vi "FGV Laser.vi"(8 "error in (no error)":errorcluster, 10 "FGV Laser Data In":T1 {"Pulse Picker Set" items=["80"=80, "40"=40, "20"=20, "10"=10, "0"=0]}, 11 "Action":T3=enum."Connect") -> (0 "error out":errorcluster, 3 "FGV Laser Data Out":T1 {"Pulse Picker Set" items=["80"=80, "40"=40, "20"=20, "10"=10, "0"=0]})   [LabVIEW 2017]
uses:
  Action Laser.ctl
  FGV Laser Data.ctl
  PulsePickerValues.ctl
  <vilib>/Instr/_visa.llb/VISA Configure Serial Port (Instr).vi
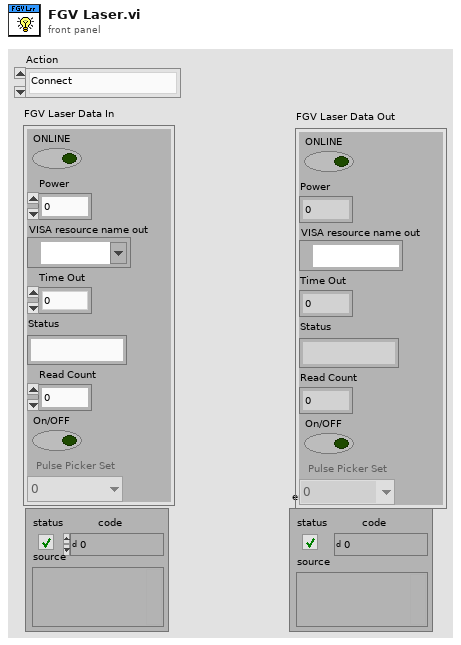
[diagram p1: front panel]
types:
  T1 = typedef "FGV Laser Data.ctl" = cluster{"ONLINE":bool, "Power":dbl, "VISA resource name out":refnum<visa-resource-name>, "Time Out":dbl, "Status":string, "Read Count":u32, "On/OFF":bool, "Pulse Picker Set":T2}
  T2 = typedef "PulsePickerValues.ctl" = u16
  T3 = typedef "Action Laser.ctl" = enum16{"Initialize", "Connect", "Disconnect", "Set Power", "Get Power", "Set Pulse Picker", "Get Pulse Picker", "Laser ON", "Laser OFF", "Read Visa"}
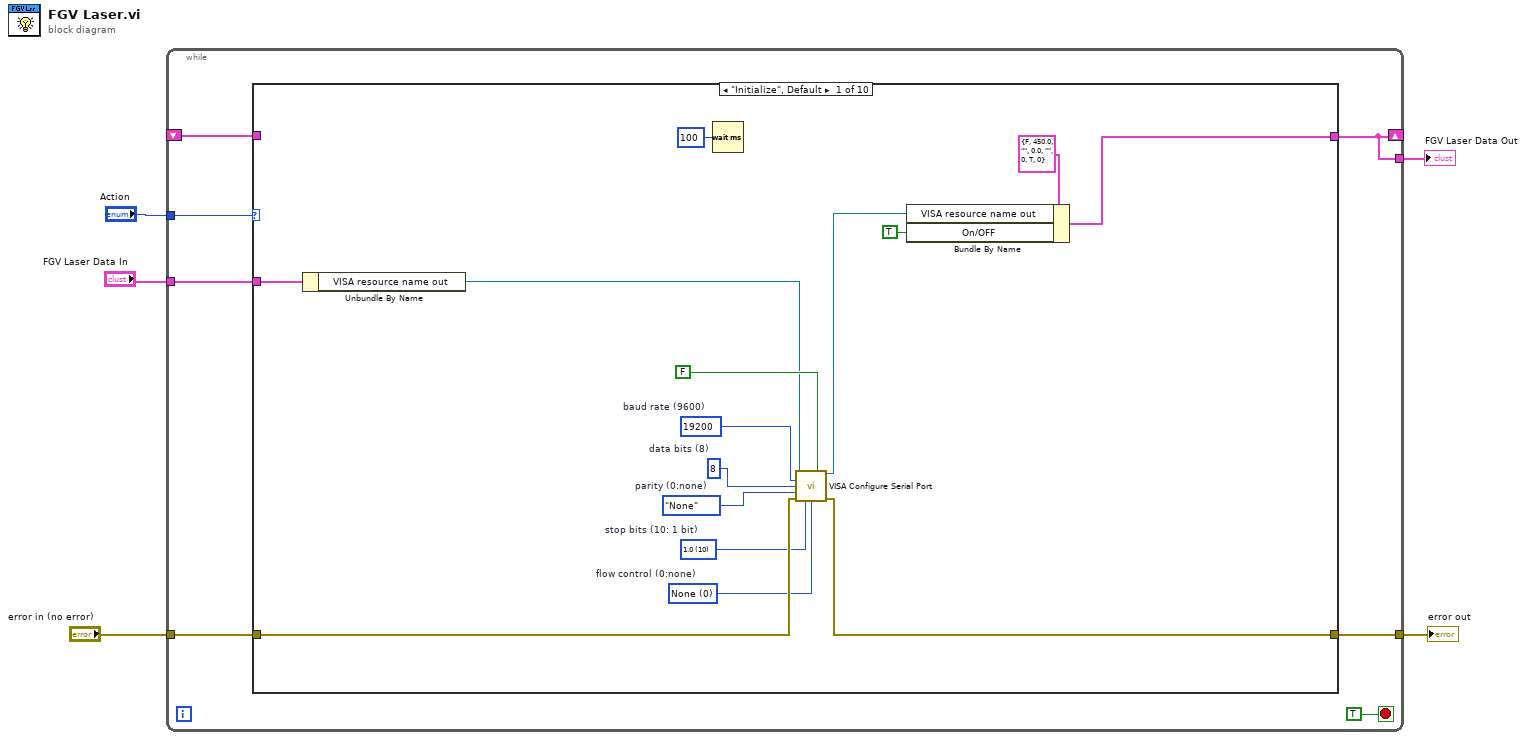
[diagram p0: block diagram]
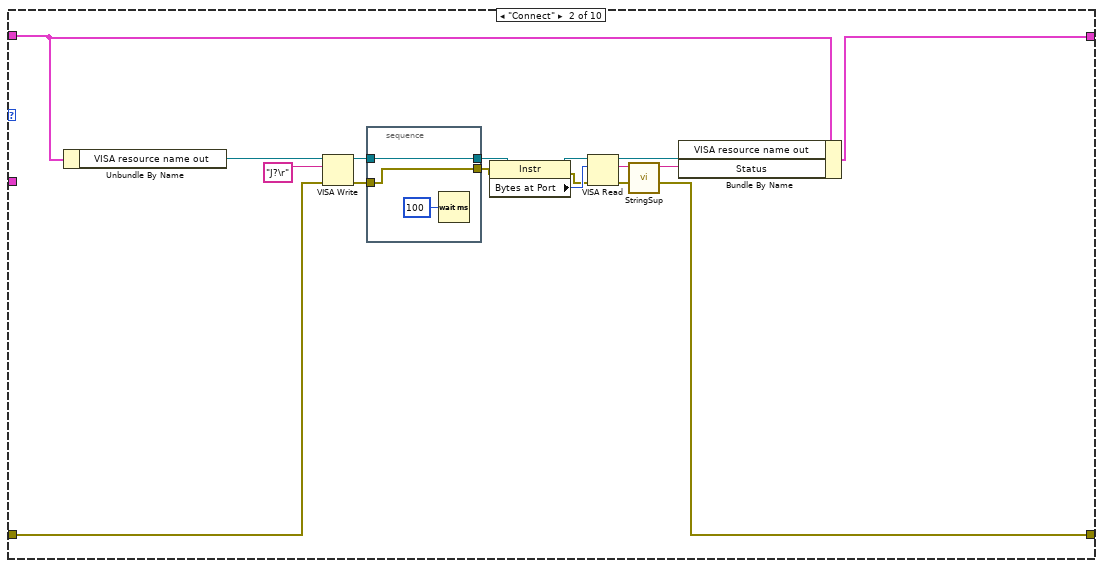
[diagram p2: hidden frame]
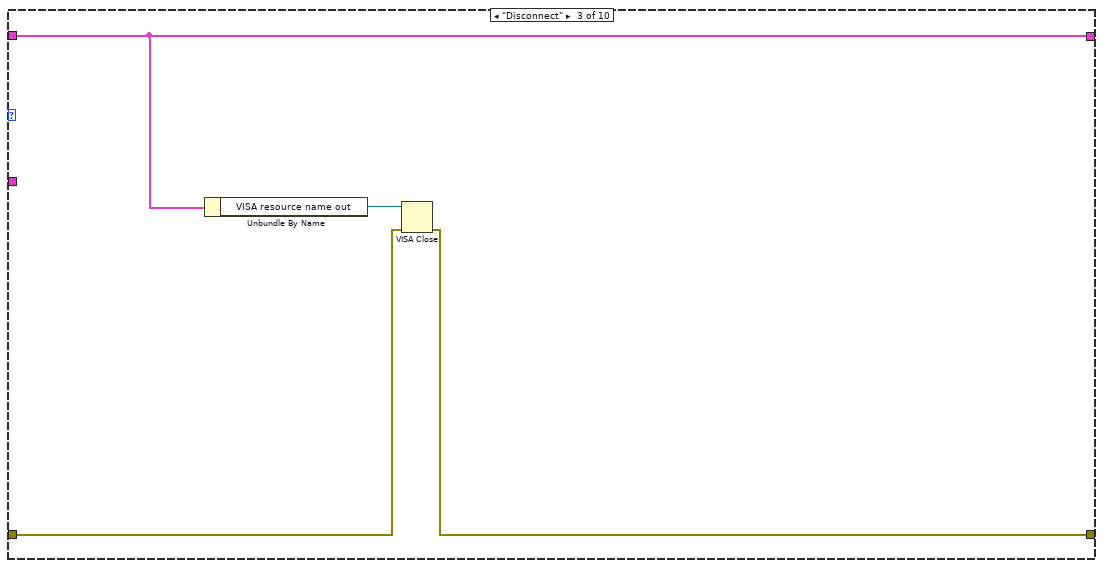
[diagram p3: hidden frame]
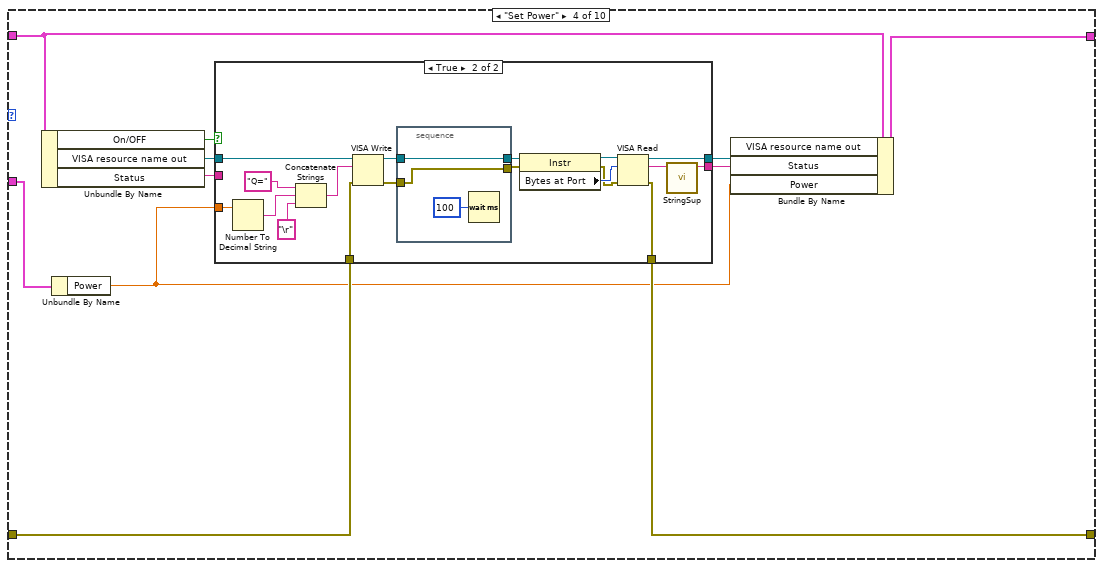
[diagram p4: hidden frame]
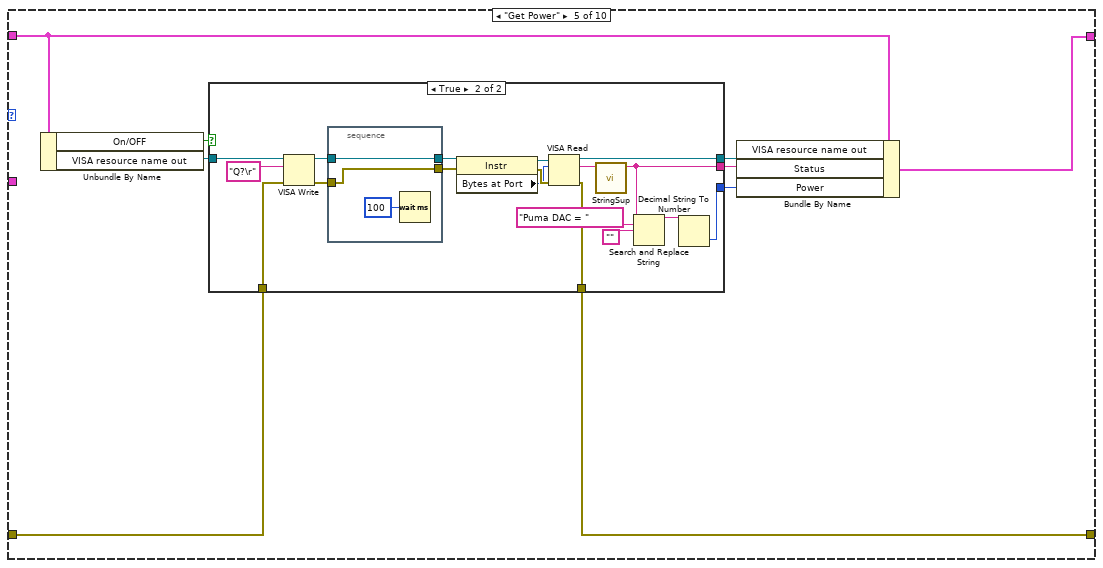
[diagram p6: hidden frame]
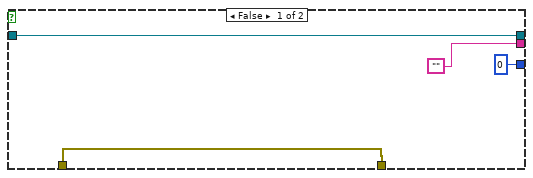
[diagram p7: hidden frame]
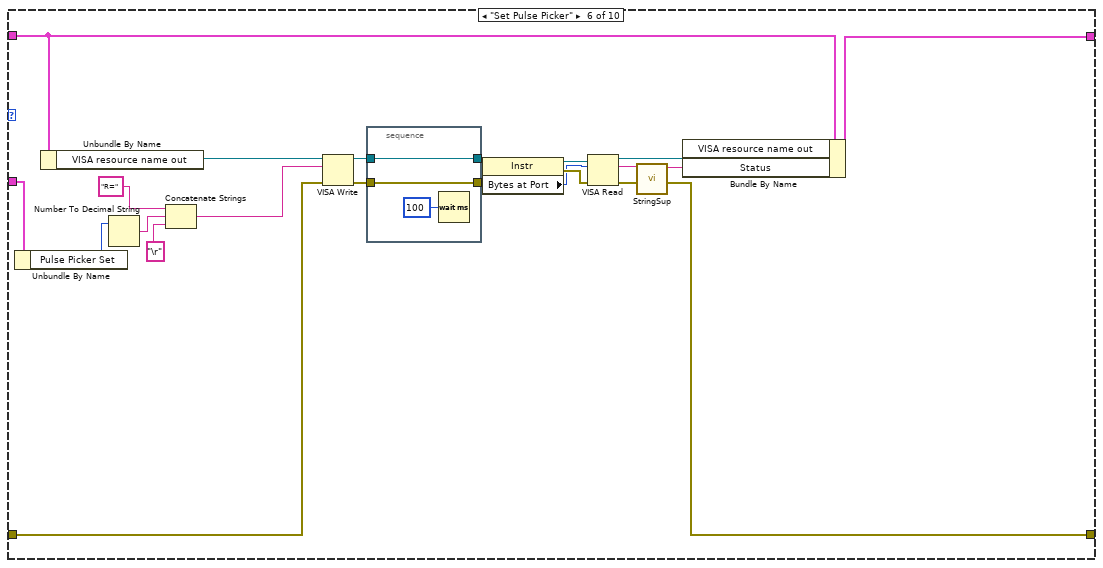
[diagram p8: hidden frame]
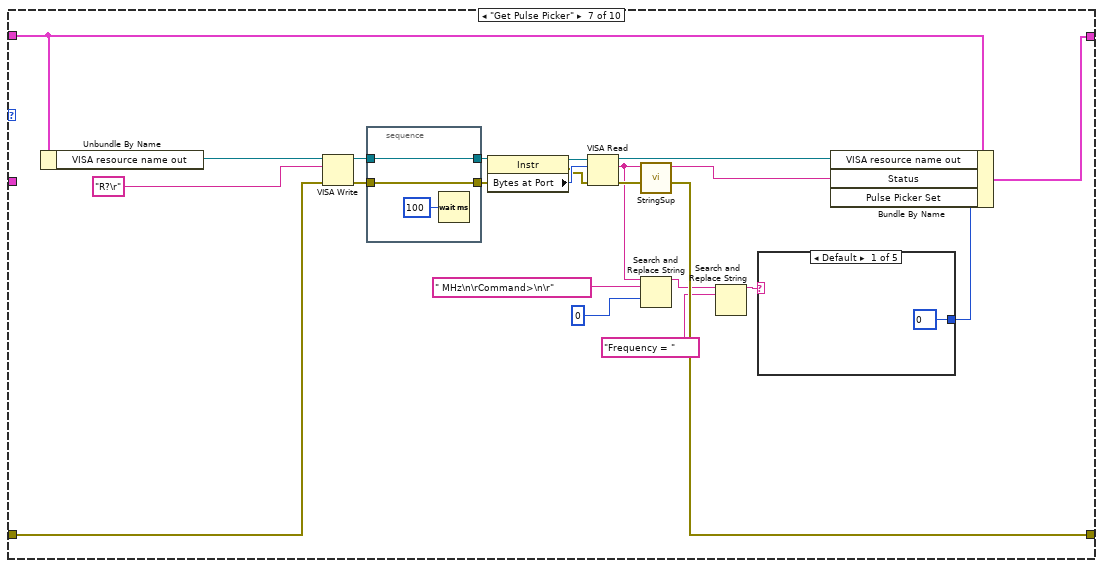
[diagram p9: hidden frame]
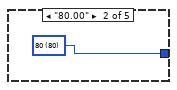
[diagram p10: hidden frame]
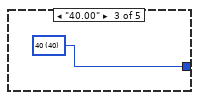
[diagram p11: hidden frame]
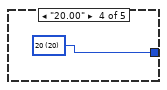
[diagram p12: hidden frame]
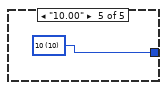
[diagram p13: hidden frame]
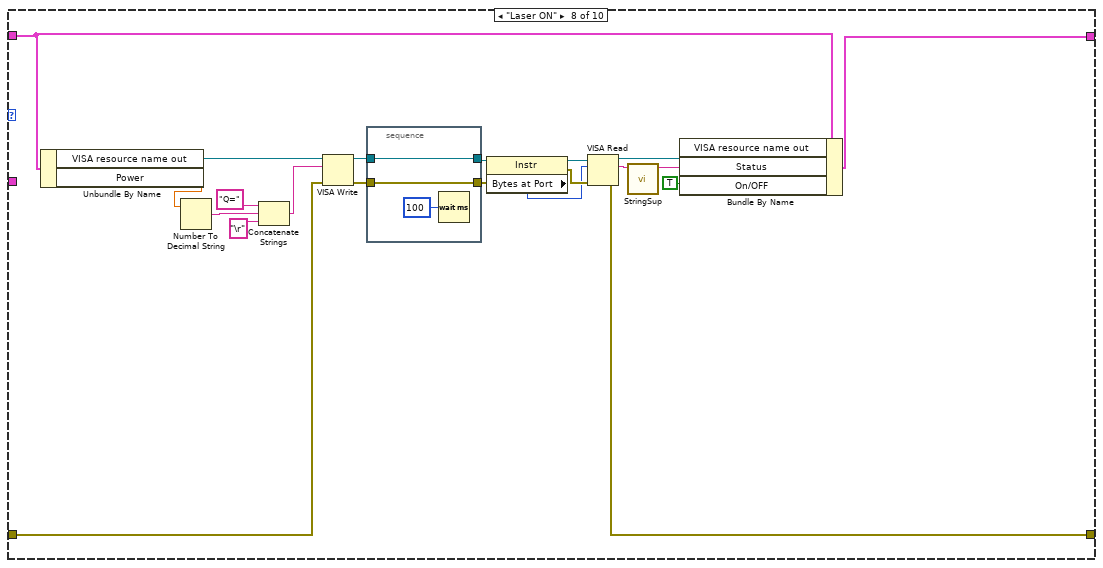
[diagram p14: hidden frame]
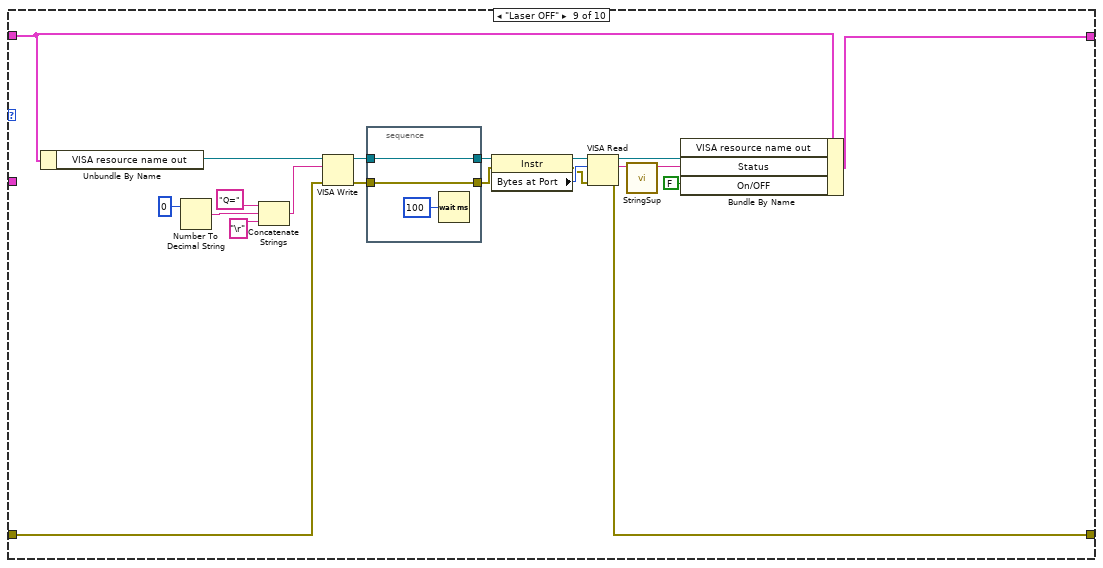
[diagram p15: hidden frame]
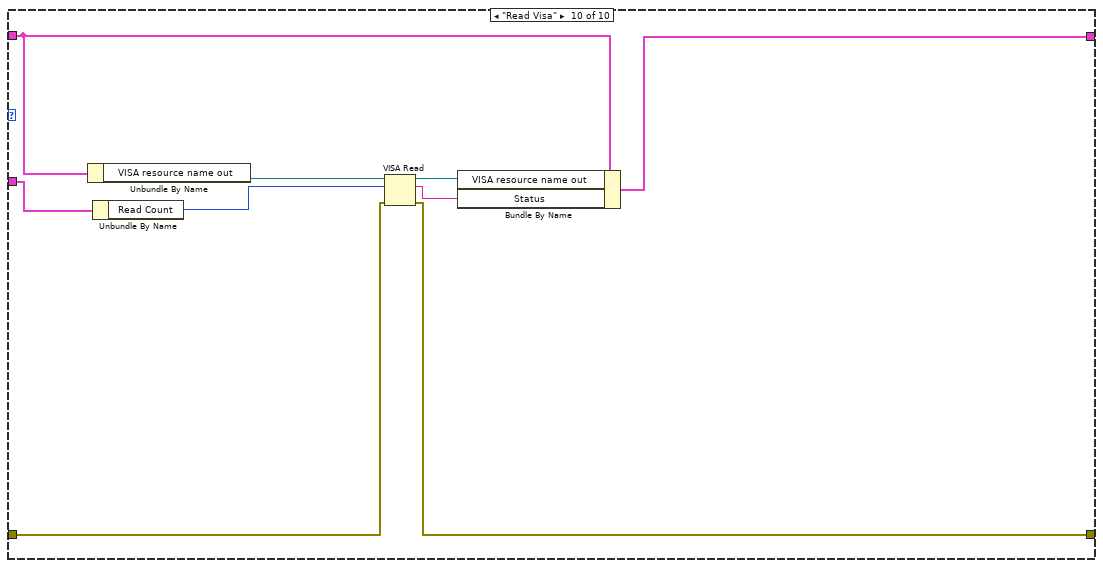
[diagram p16: hidden frame]
diagram:
  n1 = while {
    tunnel: "Action" -> [w11]
    tunnel: "error in (no error)" -> [w10]
    tunnel: [w9] -> w3
    shift-right: [w6] -> _
    shift-left: _ -> [w8]
    tunnel: "FGV Laser Data In" -> [w7]
    tunnel: [w6] -> w1
    stop <- TRUE stop-if-true
    n2 = case shown="\"Initialize\", Default" w11 {
      tunnel: [w24 w35 w47 w56 w89 w133 w158 w187 w211 w228] -> w9
      tunnel: w10 -> [w25 w42 w48 w60 w93 w139 w164 w193 w217 w229]
      tunnel: [w21 w39 w50 w58 w91 w137 w162 w191 w215 w222] -> w6
      tunnel: w8 -> [_ w40 w50 w59 w92 w138 w163 w192 w216 w225]
      tunnel: w7 -> [w23 _ _ w55 _ w132 _ _ _ w227]
      frame "Initialize", Default {
        w17 = u16 0 items=["None", "XON/XOFF", "RTS/CTS", "XON/XOFF & RTS/CTS", "DTR/DSR", "XON/XOFF & DTR/DSR"]  # flow control (0:none)
        w18 = u16 10 items=["1.0"=10, "1.5"=15, "2.0"=20]  # stop bits (10: 1 bit)
        w19 = enum16{"None", "Odd", "Even", "Mark", "Space"}."None"  # parity (0:none)
        w26 = u16 8  # data bits (8)
        w27 = u32 19200  # baud rate (9600)
        n3 = Unbundle By Name(w23) -> ("VISA resource name out"=w15:refnum<visa-resource-name>)
        n4 = Wait (ms)(milliseconds to wait=u32 100) -> ()  [unwired: 1 out]
        n5 = call-poly "VISA Configure Serial Port"("VISA resource name"=w15, "Enable Termination\nChar (T)"=FALSE ("Enable Termination\nChar (T)"), "baud rate (9600)"=w27, "data bits (8)"=w26, "parity (0:none)"=w19, "error in (no error)"=w25, "stop bits (10: 1 bit)"=w18, "flow control (0:none)"=w17) -> ("VISA resource name out"=w20:refnum<visa-resource-name>, "error out"=w24:errorcluster)  [unwired: 6 in]
        n6 = Bundle By Name(cluster=T1 {"ONLINE"=FALSE, "Power"=450.0, "VISA resource name out"="", "Time Out"=0.0, "Status"="", "Read Count"=0, "On/OFF"=TRUE, "Pulse Picker Set"=0} ("FGV Laser Data"), "VISA resource name out"=w20, "On/OFF"=TRUE) -> (w21:T1)
      }
      frame "Connect" {
        n7 = Unbundle By Name(w40) -> ("VISA resource name out"=w43:refnum<visa-resource-name>)
        n8 = VISA Write(VISA resource name=w43, write buffer="J?\r", error in (no error)=w42) -> (VISA resource name out=w37:refnum<visa-resource-name>, error out=w38:errorcluster)  [unwired: 1 out]
        n9 = stacked-sequence {
          tunnel: w38 -> [w44]
          tunnel: w37 -> [w45]
          tunnel: [w45] -> w34
          tunnel: [w44] -> w31
          frame #0 {
            n10 = Wait (ms)(milliseconds to wait=u32 100) -> ()  [unwired: 1 out]
          }
        }
        n11 = property class="Instr"(reference=w34, error in=w31) -> (reference out=w32:refnum<visa-resource-name>, error out=w30:errorcluster, "Bytes at Port"=w33:u32)
        n12 = VISA Read(VISA resource name=w32, byte count=w33, error in (no error)=w30) -> (VISA resource name out=w36:refnum<visa-resource-name>, read buffer=w29:string, error out=w35:errorcluster)  [unwired: 1 out]
        n13 = call "StringSup.vi"("String"=w29) -> ("result string"=w28:string)  [unwired: 10 in]
        n14 = Bundle By Name(cluster=w40, "VISA resource name out"=w36, "Status"=w28) -> (w39:T1)
      }
      frame "Disconnect" {
        n15 = Unbundle By Name(w50) -> ("VISA resource name out"=w49:refnum<visa-resource-name>)
        n16 = VISA Close(VISA resource name=w49, error in (no error)=w48) -> (error out=w47:errorcluster)
      }
      frame "Set Power" {
        n17 = Unbundle By Name(w59) -> ("On/OFF"=w52:bool, "VISA resource name out"=w61:refnum<visa-resource-name>, "Status"=w51:string)
        n18 = Unbundle By Name(w55) -> ("Power"=w54:dbl)
        n19 = case shown="True" w52 {
          tunnel: w61 -> [w63 w82]
          tunnel: w60 -> [w62 w81]
          tunnel: [w63 w78] -> w57
          tunnel: [w62 w77] -> w56
          tunnel: w54 -> [_ w72]
          tunnel: [w64 w65] -> w53
          tunnel: w51 -> [w64 _]
          frame False {
          }
          frame True {
            n20 = Number To Decimal String(number=w72) -> (decimal integer string=w75:string)  [unwired: 1 in]
            n21 = Concatenate Strings("Q=" ("write buffer"), w75, "\r" ("string")) -> (w73:string)
            n22 = VISA Write(VISA resource name=w82, write buffer=w73, error in (no error)=w81) -> (VISA resource name out=w79:refnum<visa-resource-name>, error out=w80:errorcluster)  [unwired: 1 out]
            n23 = stacked-sequence {
              tunnel: w80 -> [w83]
              tunnel: w79 -> [w84]
              tunnel: [w84] -> w71
              tunnel: [w83] -> w70
              frame #0 {
                n24 = Wait (ms)(milliseconds to wait=u32 100) -> ()  [unwired: 1 out]
              }
            }
            n25 = property class="Instr"(reference=w71, error in=w70) -> (reference out=w69:refnum<visa-resource-name>, error out=w67:errorcluster, "Bytes at Port"=w68:u32)
            n26 = VISA Read(VISA resource name=w69, byte count=w68, error in (no error)=w67) -> (VISA resource name out=w78:refnum<visa-resource-name>, read buffer=w66:string, error out=w77:errorcluster)  [unwired: 1 out]
            n27 = call "StringSup.vi"("String"=w66) -> ("result string"=w65:string)  [unwired: 10 in]
          }
        }
        n28 = Bundle By Name(cluster=w59, "VISA resource name out"=w57, "Status"=w53, "Power"=w54) -> (w58:T1)
      }
      frame "Get Power" {
        n29 = Unbundle By Name(w92) -> ("On/OFF"=w87:bool, "VISA resource name out"=w94:refnum<visa-resource-name>)
        n30 = case shown="True" w87 {
          tunnel: w94 -> [w98 w116]
          tunnel: w93 -> [w97 w115]
          tunnel: [w98 w112] -> w90
          tunnel: [w97 w111] -> w89
          tunnel: ["" w100] -> w88
          tunnel: [0 w99] -> w86
          frame False {
          }
          frame True {
            n31 = VISA Write(VISA resource name=w116, write buffer="Q?\r", error in (no error)=w115) -> (VISA resource name out=w113:refnum<visa-resource-name>, error out=w114:errorcluster)  [unwired: 1 out]
            n32 = stacked-sequence {
              tunnel: w114 -> [w117]
              tunnel: w113 -> [w118]
              tunnel: [w118] -> w109
              tunnel: [w117] -> w108
              frame #0 {
                n33 = Wait (ms)(milliseconds to wait=u32 100) -> ()  [unwired: 1 out]
              }
            }
            n34 = property class="Instr"(reference=w109, error in=w108) -> (reference out=w107:refnum<visa-resource-name>, error out=w106:errorcluster, "Bytes at Port"=w105:u32)
            n35 = VISA Read(VISA resource name=w107, byte count=w105, error in (no error)=w106) -> (VISA resource name out=w112:refnum<visa-resource-name>, read buffer=w104:string, error out=w111:errorcluster)  [unwired: 1 out]
            n36 = call "StringSup.vi"("String"=w104) -> ("result string"=w100:string)  [unwired: 10 in]
            n37 = Search and Replace String(input string=w100, search string="Puma DAC = ", replace string="") -> (result string=w101:string)  [unwired: 5 in, 3 out]
            n38 = Decimal String To Number(string=w101) -> (number=w99:i32)  [unwired: 2 in, 1 out]
          }
        }
        n39 = Bundle By Name(cluster=w92, "VISA resource name out"=w90, "Status"=w88, "Power"=w86) -> (w91:T1)
      }
      frame "Set Pulse Picker" {
        n40 = Unbundle By Name(w132) -> ("Pulse Picker Set"=w131:T2)
        n41 = Unbundle By Name(w138) -> ("VISA resource name out"=w140:refnum<visa-resource-name>)
        n42 = Number To Decimal String(number=w131) -> (decimal integer string=w129:string)  [unwired: 1 in]
        n43 = Concatenate Strings("R=" ("write buffer"), w129, "\r" ("string")) -> (w127:string)
        n44 = VISA Write(VISA resource name=w140, write buffer=w127, error in (no error)=w139) -> (VISA resource name out=w135:refnum<visa-resource-name>, error out=w136:errorcluster)  [unwired: 1 out]
        n45 = stacked-sequence {
          tunnel: w136 -> [w141]
          tunnel: w135 -> [w142]
          tunnel: [w142] -> w126
          tunnel: [w141] -> w125
          frame #0 {
            n46 = Wait (ms)(milliseconds to wait=u32 100) -> ()  [unwired: 1 out]
          }
        }
        n47 = property class="Instr"(reference=w126, error in=w125) -> (reference out=w124:refnum<visa-resource-name>, error out=w123:errorcluster, "Bytes at Port"=w122:u32)
        n48 = VISA Read(VISA resource name=w124, byte count=w122, error in (no error)=w123) -> (VISA resource name out=w134:refnum<visa-resource-name>, read buffer=w121:string, error out=w133:errorcluster)  [unwired: 1 out]
        n49 = call "StringSup.vi"("String"=w121) -> ("result string"=w120:string)  [unwired: 10 in]
        n50 = Bundle By Name(cluster=w138, "VISA resource name out"=w134, "Status"=w120) -> (w137:T1)
      }
      frame "Get Pulse Picker" {
        n51 = Unbundle By Name(w163) -> ("VISA resource name out"=w165:refnum<visa-resource-name>)
        n52 = VISA Write(VISA resource name=w165, write buffer="R?\r", error in (no error)=w164) -> (VISA resource name out=w160:refnum<visa-resource-name>, error out=w161:errorcluster)  [unwired: 1 out]
        n53 = stacked-sequence {
          tunnel: w161 -> [w171]
          tunnel: w160 -> [w172]
          tunnel: [w172] -> w152
          tunnel: [w171] -> w151
          frame #0 {
            n54 = Wait (ms)(milliseconds to wait=u32 100) -> ()  [unwired: 1 out]
          }
        }
        n55 = property class="Instr"(reference=w152, error in=w151) -> (reference out=w150:refnum<visa-resource-name>, error out=w148:errorcluster, "Bytes at Port"=w149:u32)
        n56 = VISA Read(VISA resource name=w150, byte count=w149, error in (no error)=w148) -> (VISA resource name out=w159:refnum<visa-resource-name>, read buffer=w147:string, error out=w158:errorcluster)  [unwired: 1 out]
        n57 = call "StringSup.vi"("String"=w147) -> ("result string"=w146:string)  [unwired: 10 in]
        n58 = Search and Replace String(input string=w147, search string=" MHz\n\rCommand>\n\r" ("substring (\"\")"), offset=0 ("offset (0)")) -> (result string=w155:string)  [unwired: 5 in, 3 out]
        n59 = Search and Replace String(input string=w155, search string="Frequency = ") -> (result string=w145:string)  [unwired: 6 in, 3 out]
        n60 = case shown="Default" w145 {
          tunnel: [w166 w167 w168 w169 w170] -> w144
          frame Default {
            w166 = T2 0 items=["80"=80, "40"=40, "20"=20, "10"=10, ""=0] ("Pulse Picker Set")
          }
          frame "80.00" {
            w167 = T2 80 items=["80"=80, "40"=40, "20"=20, "10"=10, ""=0] ("Pulse Picker Set")
          }
          frame "40.00" {
            w168 = T2 40 items=["80"=80, "40"=40, "20"=20, "10"=10, ""=0] ("Pulse Picker Set")
          }
          frame "20.00" {
            w169 = T2 20 items=["80"=80, "40"=40, "20"=20, "10"=10, ""=0] ("Pulse Picker Set")
          }
          frame "10.00" {
            w170 = T2 10 items=["80"=80, "40"=40, "20"=20, "10"=10, ""=0] ("Pulse Picker Set")
          }
        }
        n61 = Bundle By Name(cluster=w163, "VISA resource name out"=w159, "Status"=w146, "Pulse Picker Set"=w144) -> (w162:T1)
      }
      frame "Laser ON" {
        n62 = Unbundle By Name(w192) -> ("VISA resource name out"=w194:refnum<visa-resource-name>, "Power"=w182:dbl)
        n63 = Number To Decimal String(number=w182) -> (decimal integer string=w185:string)  [unwired: 1 in]
        n64 = Concatenate Strings("Q=" ("write buffer"), w185, "\r" ("string")) -> (w183:string)
        n65 = VISA Write(VISA resource name=w194, write buffer=w183, error in (no error)=w193) -> (VISA resource name out=w189:refnum<visa-resource-name>, error out=w190:errorcluster)  [unwired: 1 out]
        n66 = stacked-sequence {
          tunnel: w190 -> [w195]
          tunnel: w189 -> [w196]
          tunnel: [w196] -> w181
          tunnel: [w195] -> w180
          frame #0 {
            n67 = Wait (ms)(milliseconds to wait=u32 100) -> ()  [unwired: 1 out]
          }
        }
        n68 = property class="Instr"(reference=w181, error in=w180) -> (reference out=w179:refnum<visa-resource-name>, error out=w178:errorcluster, "Bytes at Port"=w177:u32)
        n69 = VISA Read(VISA resource name=w179, byte count=w177, error in (no error)=w178) -> (VISA resource name out=w188:refnum<visa-resource-name>, read buffer=w176:string, error out=w187:errorcluster)  [unwired: 1 out]
        n70 = call "StringSup.vi"("String"=w176) -> ("result string"=w175:string)  [unwired: 10 in]
        n71 = Bundle By Name(cluster=w192, "VISA resource name out"=w188, "Status"=w175, "On/OFF"=TRUE) -> (w191:T1)
      }
      frame "Laser OFF" {
        n72 = Unbundle By Name(w216) -> ("VISA resource name out"=w218:refnum<visa-resource-name>)
        n73 = Number To Decimal String(number=0) -> (decimal integer string=w209:string)  [unwired: 1 in]
        n74 = Concatenate Strings("Q=" ("write buffer"), w209, "\r" ("string")) -> (w207:string)
        n75 = VISA Write(VISA resource name=w218, write buffer=w207, error in (no error)=w217) -> (VISA resource name out=w213:refnum<visa-resource-name>, error out=w214:errorcluster)  [unwired: 1 out]
        n76 = stacked-sequence {
          tunnel: w214 -> [w219]
          tunnel: w213 -> [w220]
          tunnel: [w220] -> w205
          tunnel: [w219] -> w204
          frame #0 {
            n77 = Wait (ms)(milliseconds to wait=u32 100) -> ()  [unwired: 1 out]
          }
        }
        n78 = property class="Instr"(reference=w205, error in=w204) -> (reference out=w203:refnum<visa-resource-name>, error out=w201:errorcluster, "Bytes at Port"=w202:u32)
        n79 = VISA Read(VISA resource name=w203, byte count=w202, error in (no error)=w201) -> (VISA resource name out=w212:refnum<visa-resource-name>, read buffer=w200:string, error out=w211:errorcluster)  [unwired: 1 out]
        n80 = call "StringSup.vi"("String"=w200) -> ("result string"=w199:string)  [unwired: 10 in]
        n81 = Bundle By Name(cluster=w216, "VISA resource name out"=w212, "Status"=w199, "On/OFF"=FALSE) -> (w215:T1)
      }
      frame "Read Visa" {
        n82 = Unbundle By Name(w225) -> ("VISA resource name out"=w230:refnum<visa-resource-name>)
        n83 = Unbundle By Name(w227) -> ("Read Count"=w226:u32)
        n84 = VISA Read(VISA resource name=w230, byte count=w226, error in (no error)=w229) -> (VISA resource name out=w224:refnum<visa-resource-name>, read buffer=w223:string, error out=w228:errorcluster)  [unwired: 1 out]
        n85 = Bundle By Name(cluster=w225, "VISA resource name out"=w224, "Status"=w223) -> (w222:T1)
      }
    }
  }
  "error out" <- w3
  "FGV Laser Data Out" <- w1
